vi "Voltage vs Signal_Data Engine_V1.vi"(2 "Control Signal In (-1~1)":dbl[](array[numeric]), 3 "Voltage in (0~Max. Vol.)":dbl[](array[numeric]), 4 "DM #":u16(ring) items=["Lower", "Upper"]) -> (0 "Voltage Out (0~Max. Vol.)":dbl[](array[numeric]), 1 "Control Signal Out (-1~1)":dbl[](array[numeric]))   [LabVIEW 2014]
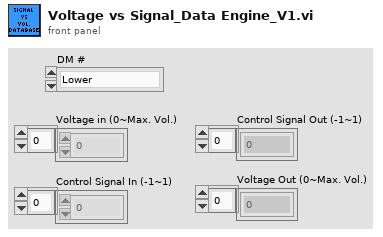
[diagram p1: front panel]
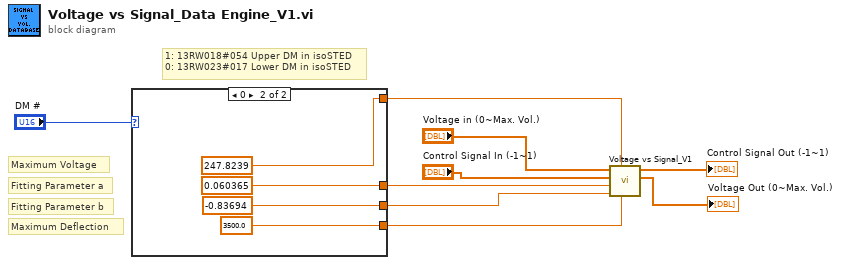
[diagram p0: block diagram]
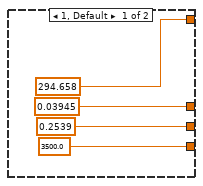
[diagram p2: hidden frame]
diagram:
  # "1: 13RW018#054 Upper DM in isoSTED\n0: 13RW023#017 Lower DM in isoSTED"
  # "Maximum Deflection"
  # "Fitting Parameter b"
  # "Fitting Parameter a"
  # "Maximum Voltage"
  n1 = case shown="0" "DM #" {
    tunnel: [294.658 247.8239] -> w8
    tunnel: [3500.0 3500.0] -> w7
    tunnel: [0.03945 0.060365] -> w6
    tunnel: [0.2539 -0.83694] -> w5
    frame 1, Default {
    }
    frame 0 {
    }
  }
  n2 = call "Voltage vs Signal_V1.vi"("Maximum Deflection"=w7, "Maximum Voltage"=w8, "b"=w5, "a"=w6, "Control Signal In (-1~1)"="Control Signal In (-1~1)", "Voltage in (0~Max. Vol.)"="Voltage in (0~Max. Vol.)") -> ("Voltage Out (0~Max. Vol.)"=→"Voltage Out (0~Max. Vol.)":dbl[], "Control Signal Out (-1~1)"=→"Control Signal Out (-1~1)":dbl[])  [unwired: 4 in]
